vi "FormMain.vi"() -> ()   [LabVIEW 2013]
uses:
  S7Ref.vi
  resultShow.vi
panel:
  out "userStatus":string
  out "productsName 2":string
  out "takesTime":string
  out "rigStatus":string="提示信息"
  out "connectionMode":string
  out "productsName":string
  out "userName":string
  in  "VI引用句柄":refnum<vi>
  in  "复位":bool
  out "上序状态":string
  out "检具15":bool=TRUE
  out "扫码":bool
  in  "壳体码":string
  in  "countLeft":u32
  out "检具7":bool
  out "检具8":bool=TRUE
  in  "判定设定 2":string[][](table)
  in  "参数设定 2":string[][](table)
  out "表格控件":string[][](table)
  out "FFT范围 2":string[][](table)
  out "压力损失":bool
  out "外泄漏":bool
  out "检具9":bool
  out "检具10":bool=TRUE
  out "检具2":bool
  out "输出扭矩":dbl caption="数值 24" format="%.1f Nm"
  in  "打开按钮":bool
  in  "自动":bool
  out "检具1":bool=TRUE
  out "检具3":bool
  out "检具4":bool
  out "检具5":bool
  out "检具6":bool
  # "出厂检验台"
  # "步骤"
  # "完成计数："
  # "用时："
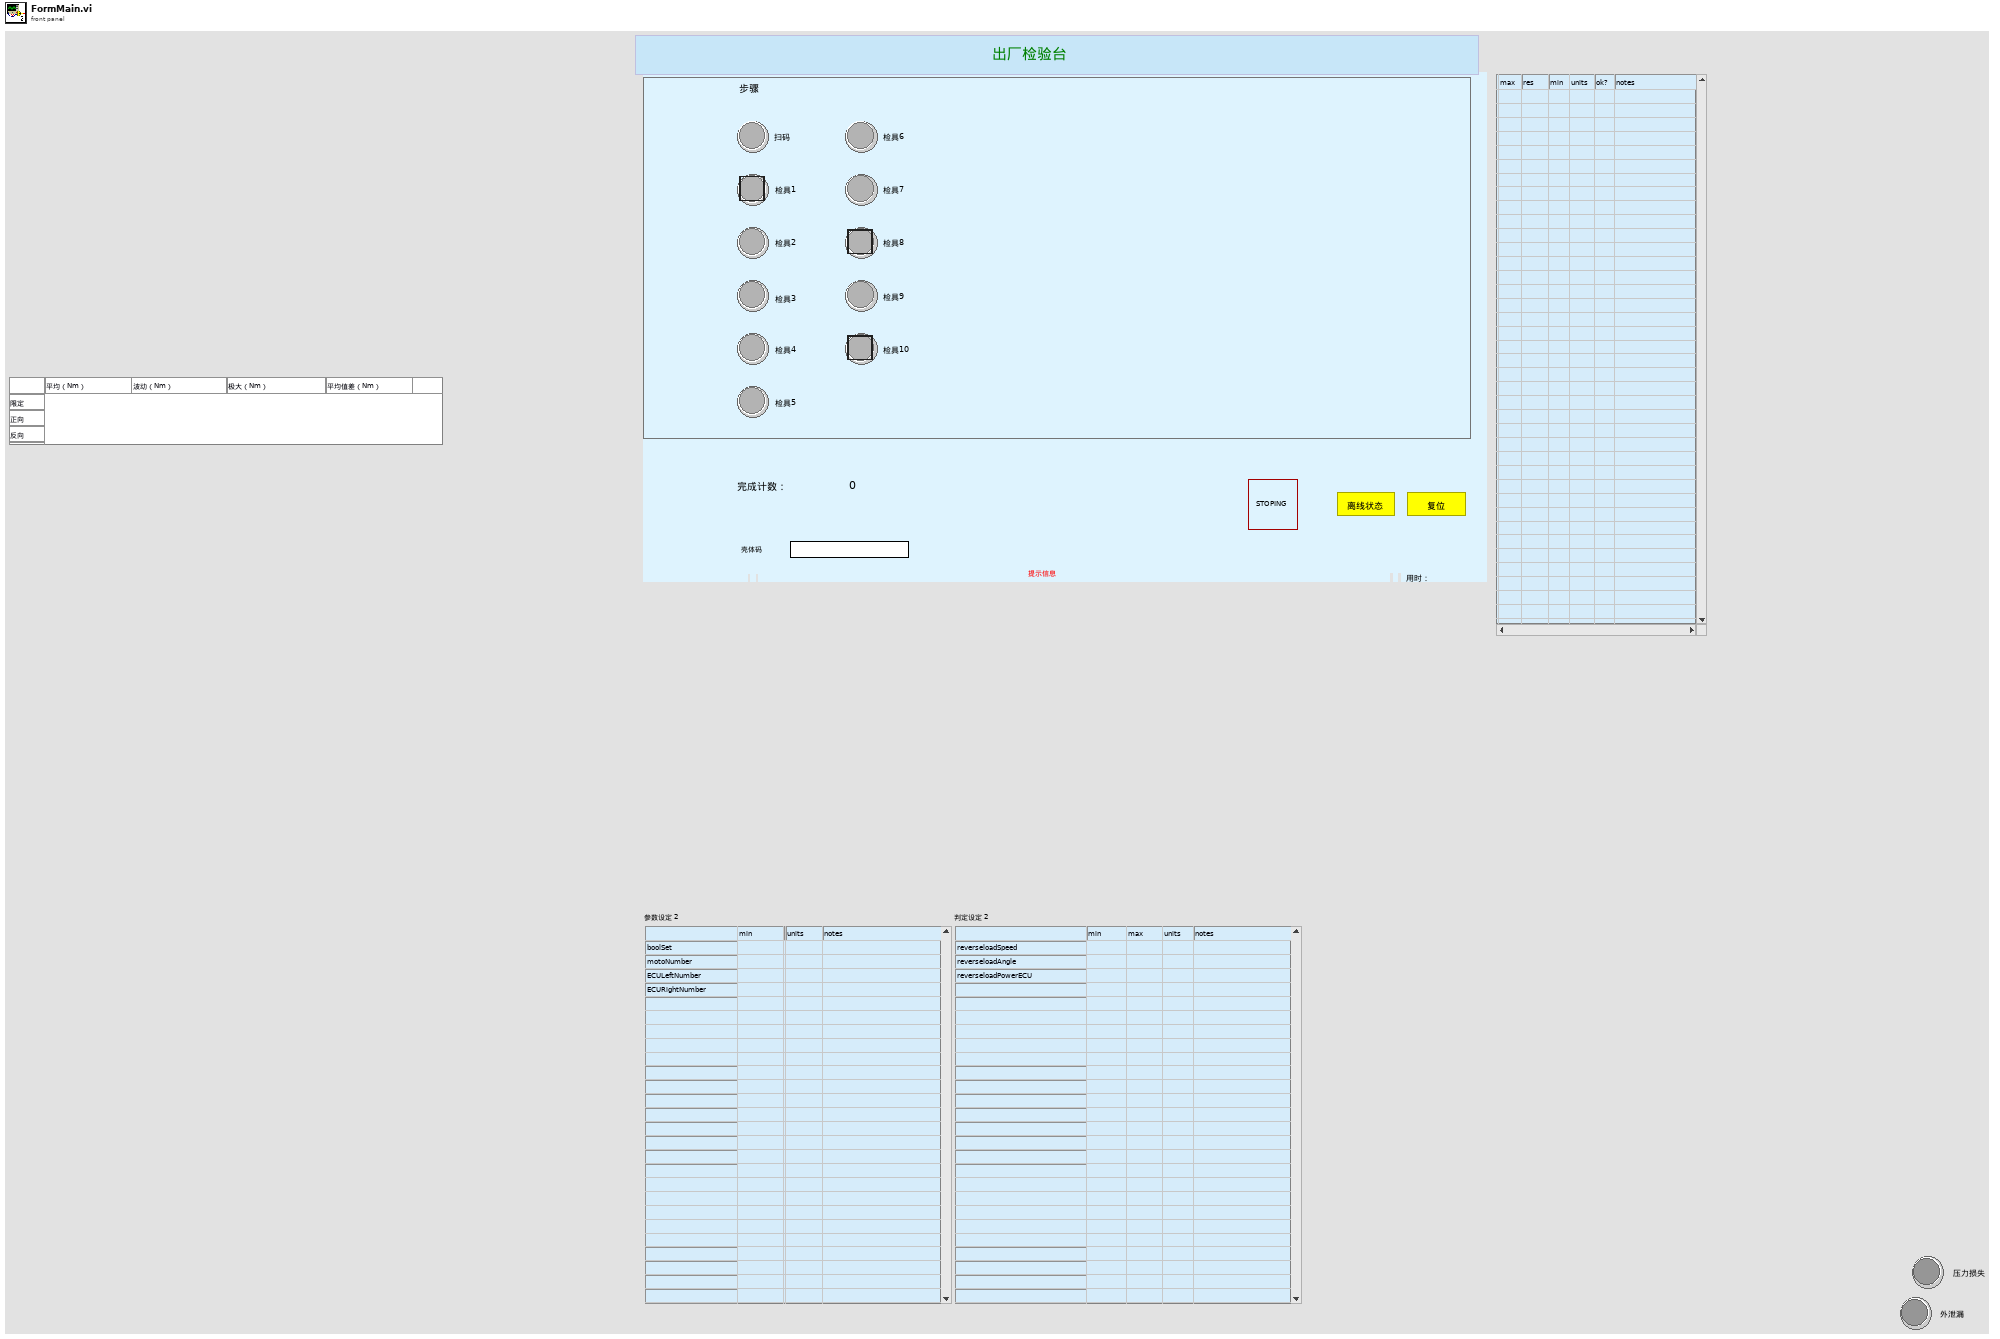
[diagram p1: front panel]
types:
  T1 = enum32{"Invalid", "Standard", "Closed", "Hidden", "Minimized", "Maximized"}
  T2 = cluster{"takesTime":refnum<vi>, "userStatus":refnum<vi>, "userName":refnum<vi>, "connectionMode":refnum<vi>, "productsName":refnum<vi>, "rigStatus":refnum<vi>, "壳体码":refnum<vi>, "上序状态":refnum<vi>}
  T3 = cluster{"userCode":string, "userName":string, "userStatus":string, "connectionMode":string}
  T4 = cluster{"Boolean array[0]":bool, "Boolean array[1]":bool, "Boolean array[2]":bool, "Boolean array[3]":bool, "Boolean array[4]":bool, "Boolean array[5]":bool, "Boolean array[6]":bool, "Boolean array[7]":bool, "Boolean array[8]":bool}
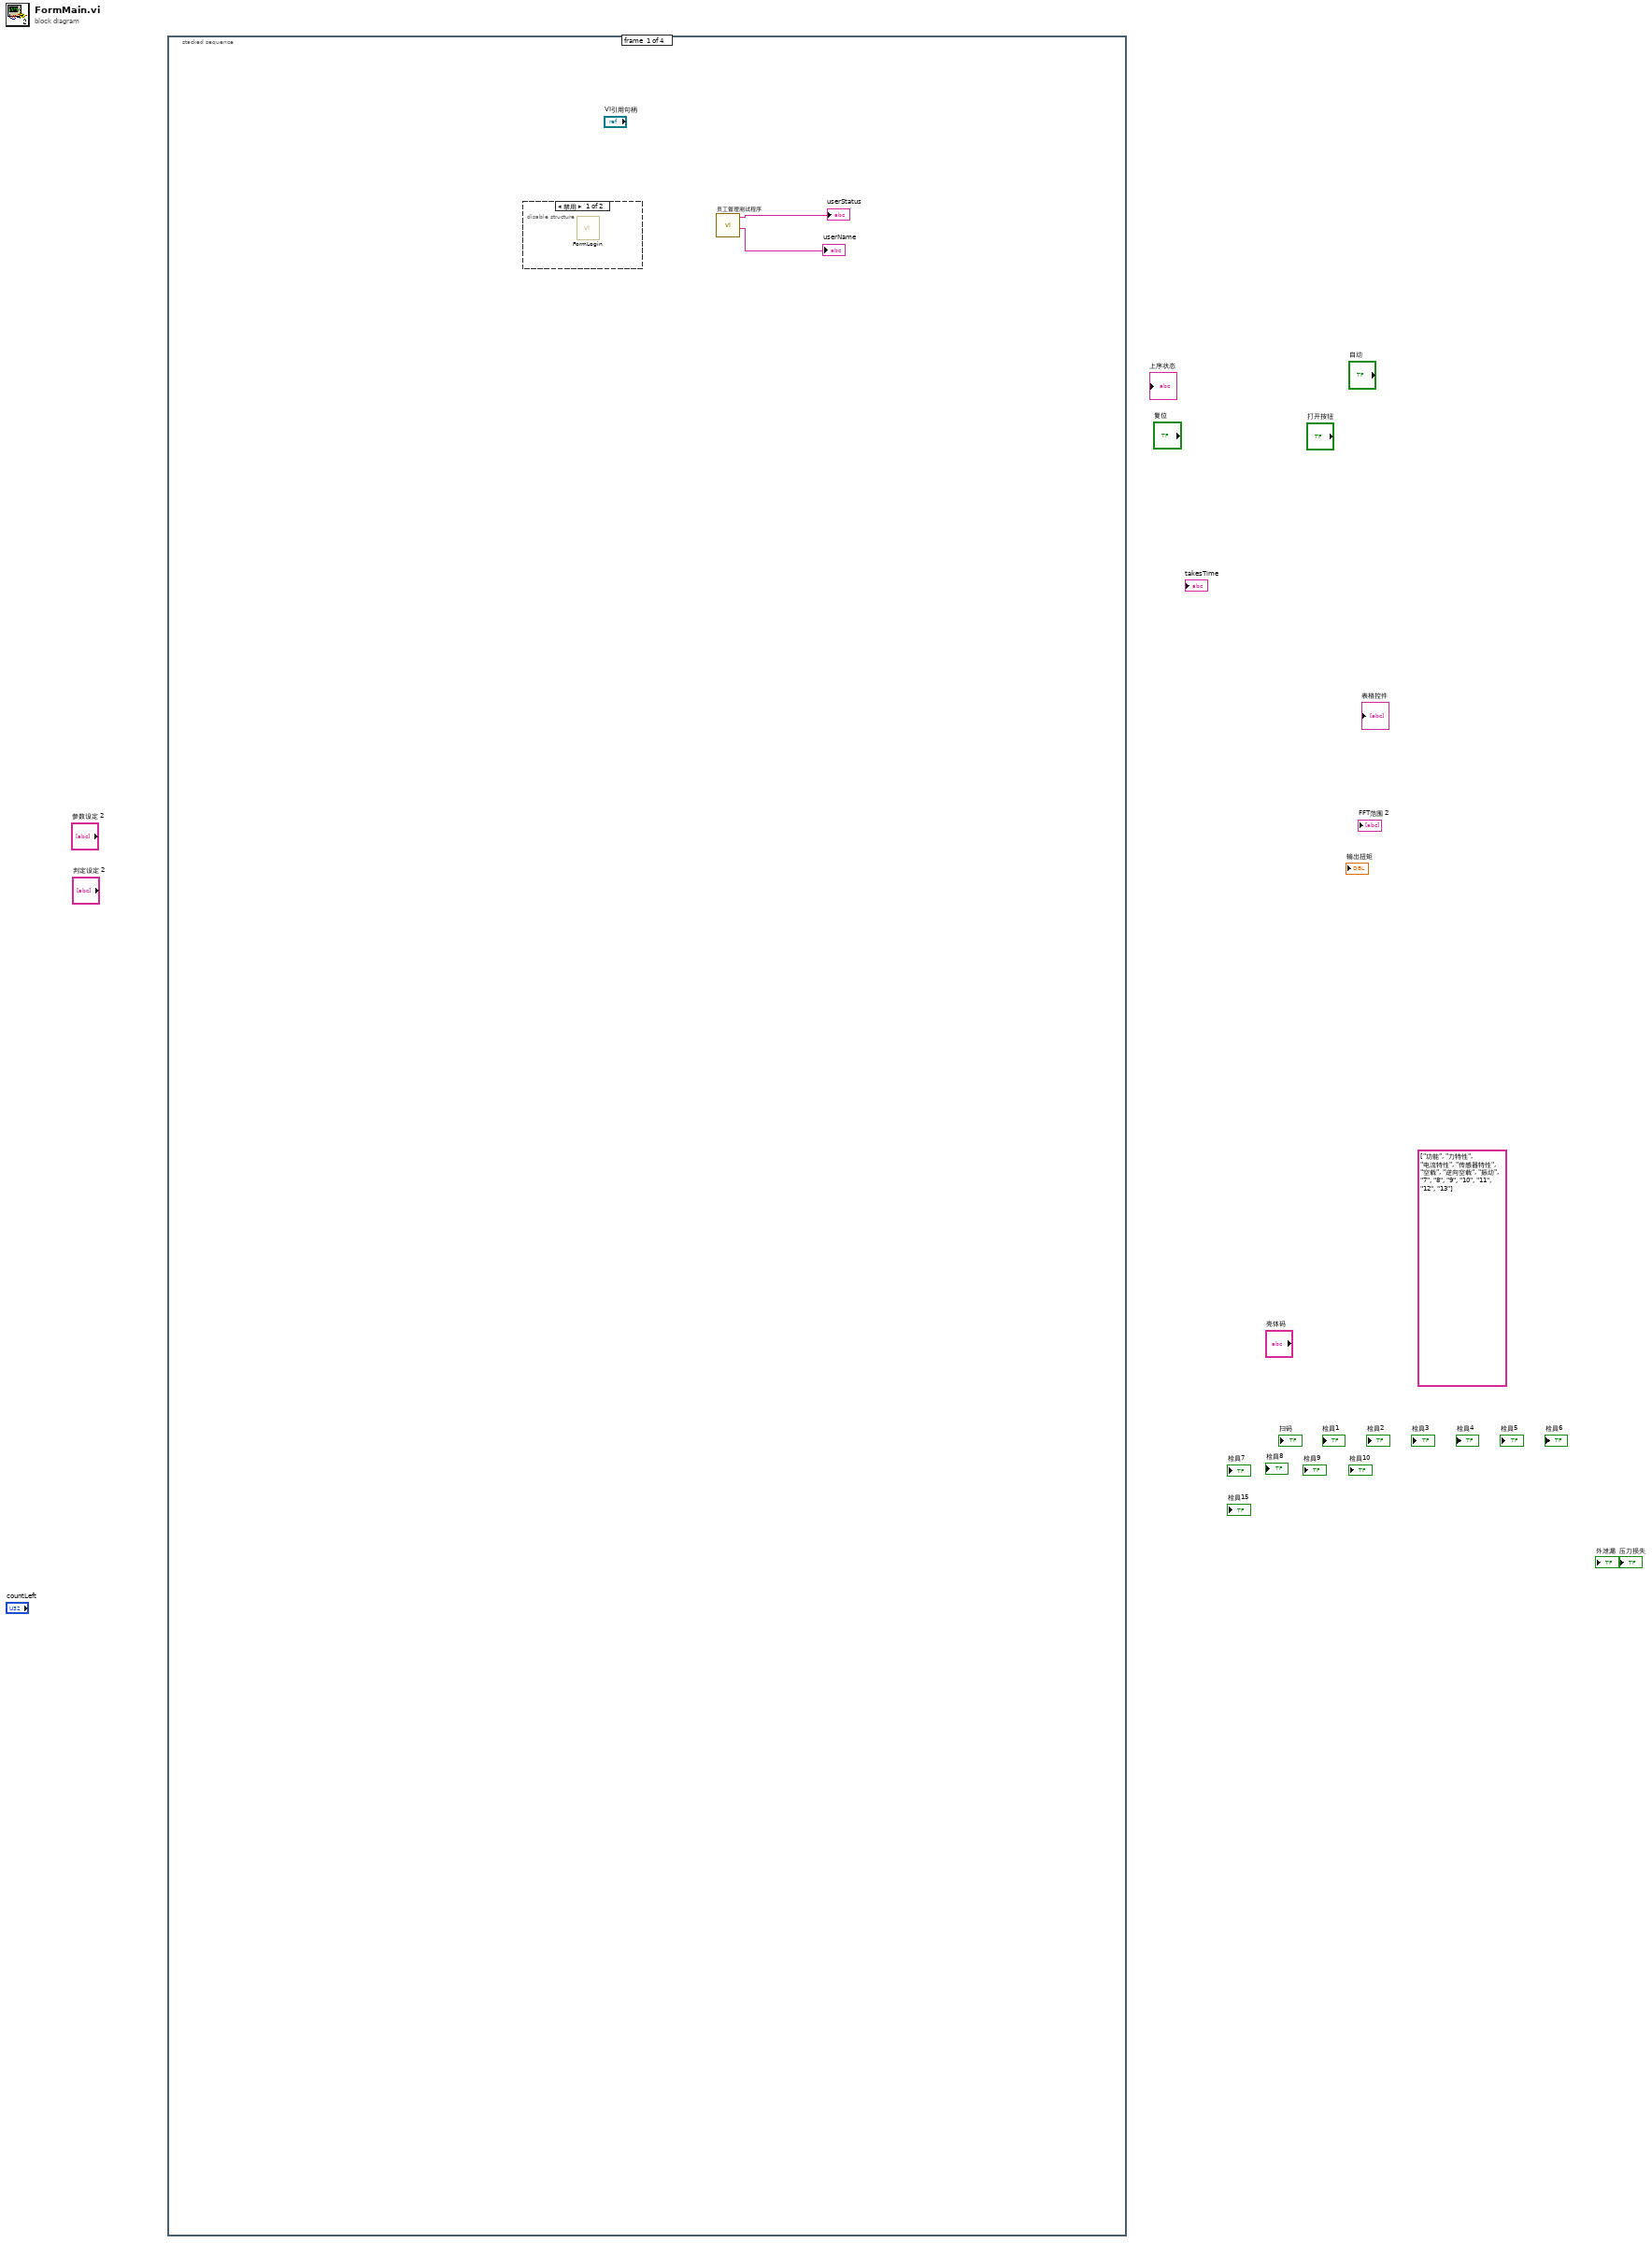
[diagram p0: block diagram]
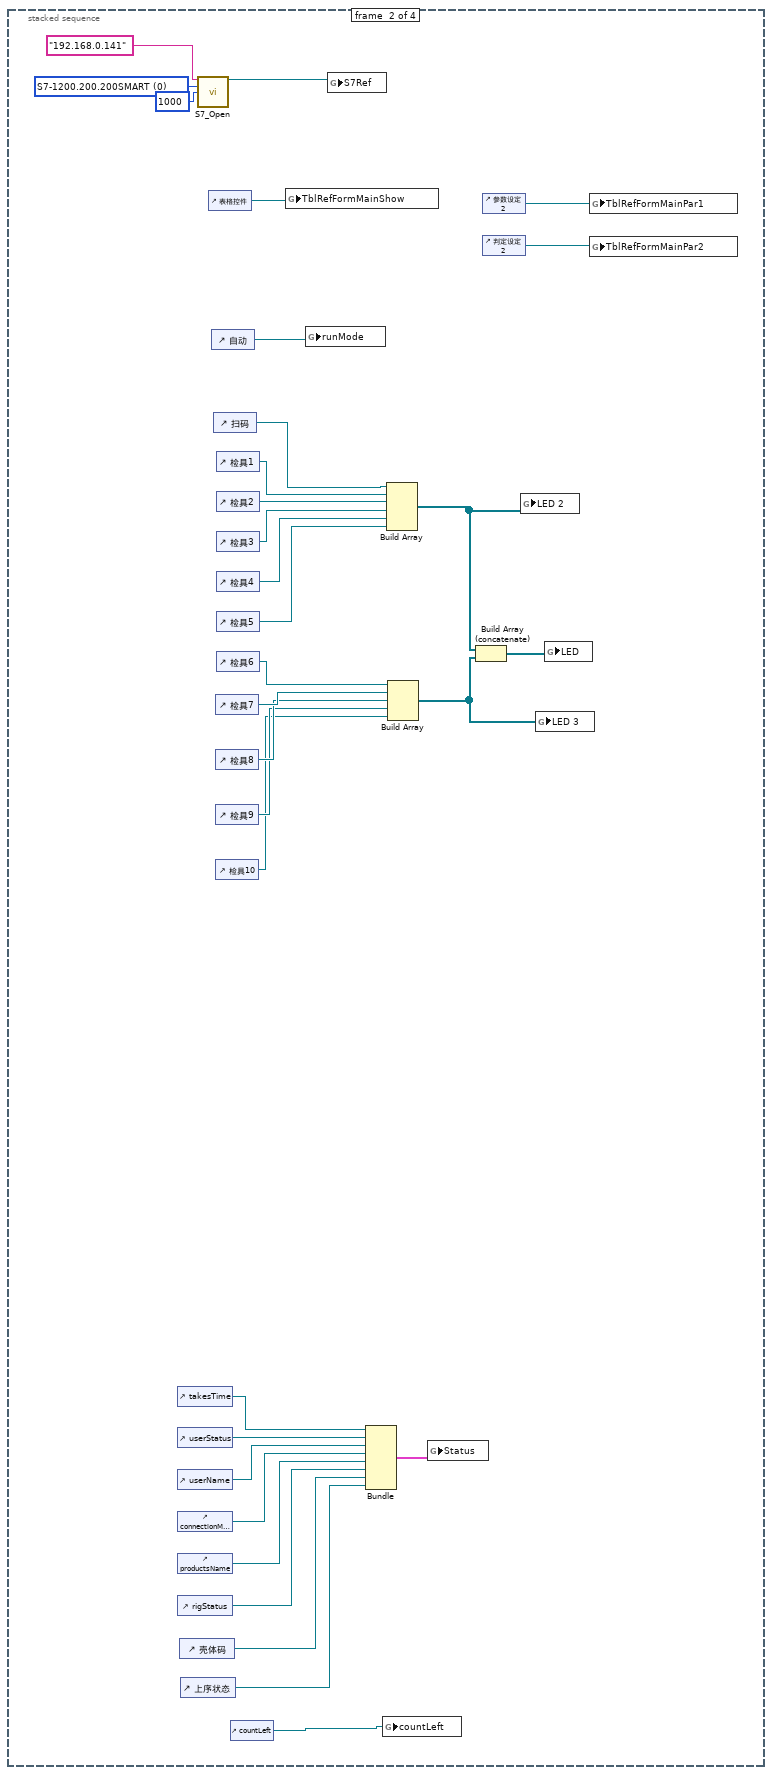
[diagram p3: hidden frame]
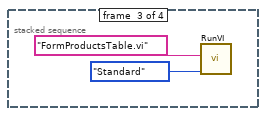
[diagram p4: hidden frame]
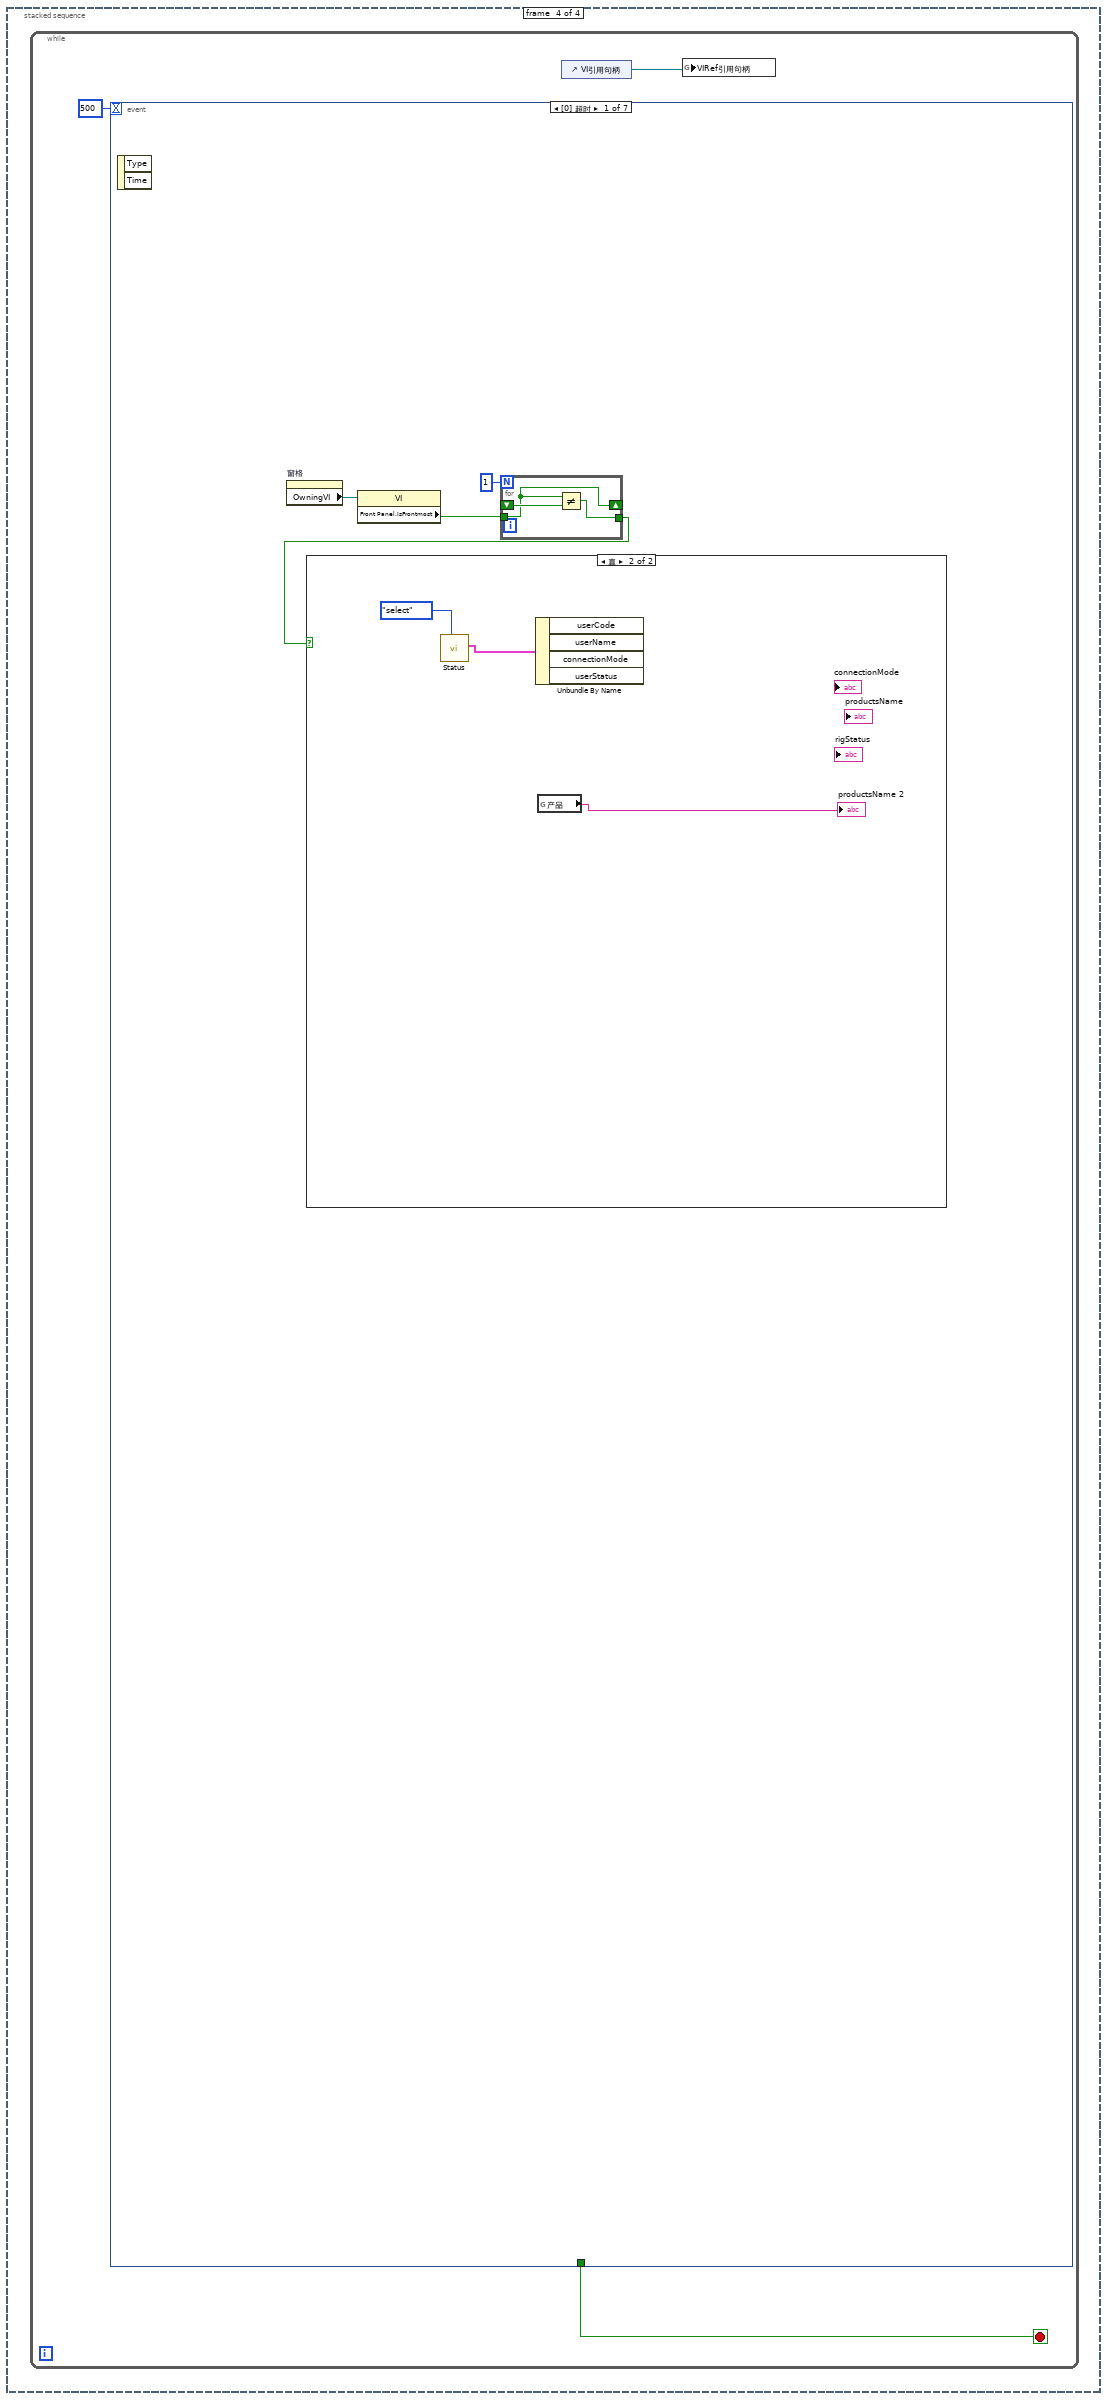
[diagram p5: hidden frame]
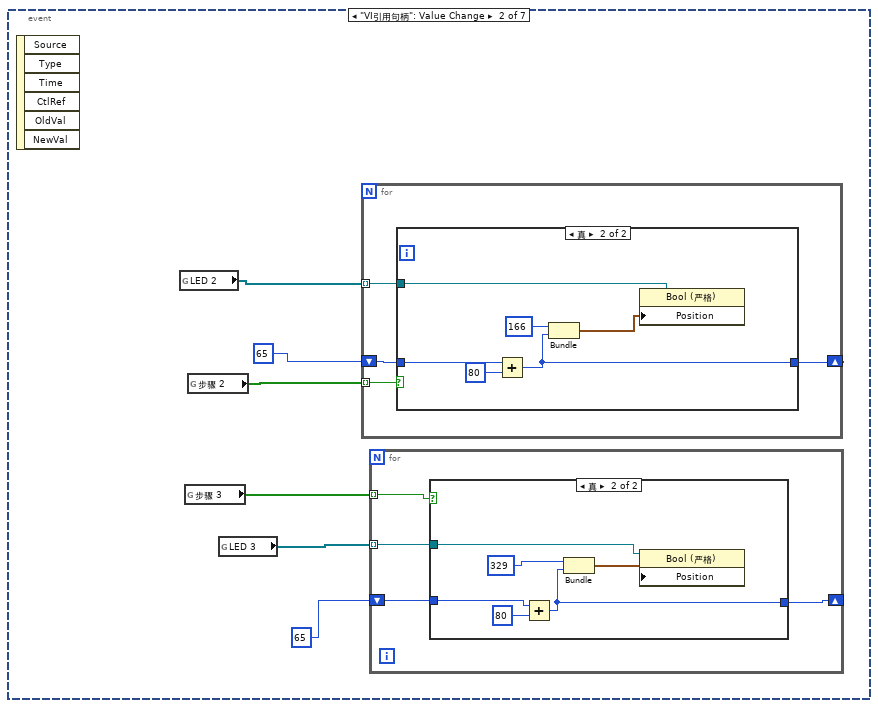
[diagram p7: hidden frame]
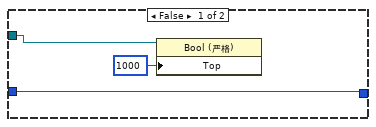
[diagram p8: hidden frame]
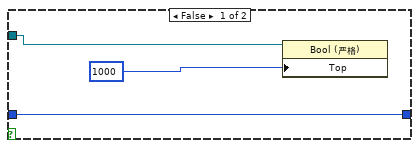
[diagram p9: hidden frame]
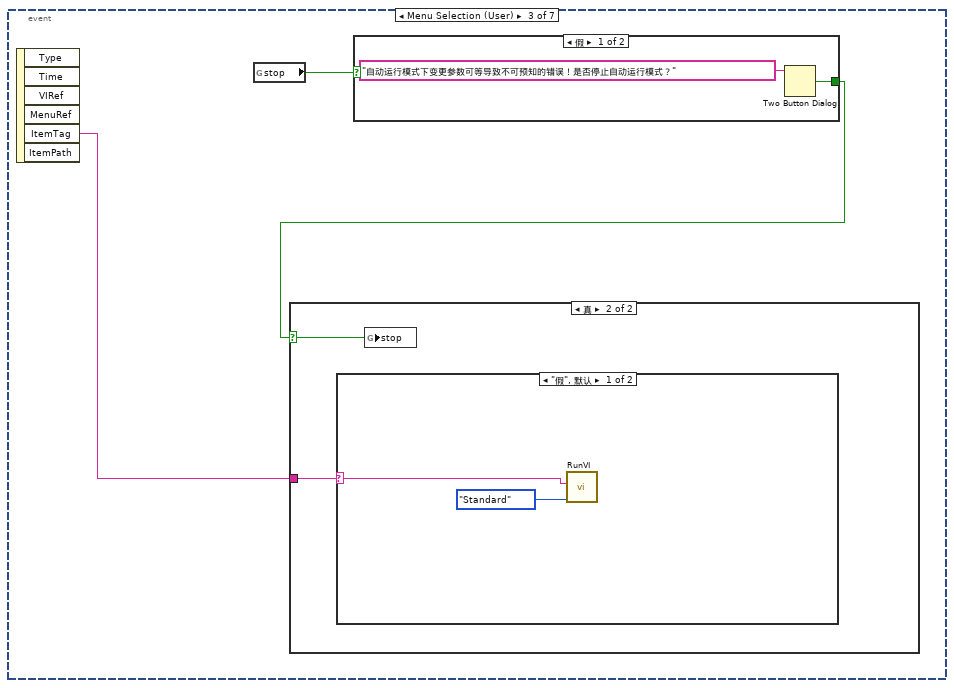
[diagram p10: hidden frame]
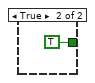
[diagram p11: hidden frame]
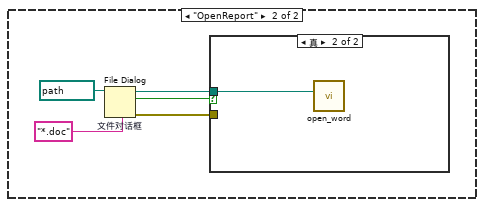
[diagram p13: hidden frame]
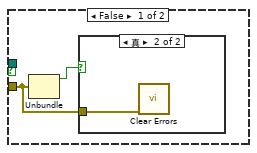
[diagram p14: hidden frame]
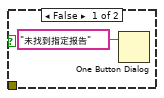
[diagram p15: hidden frame]
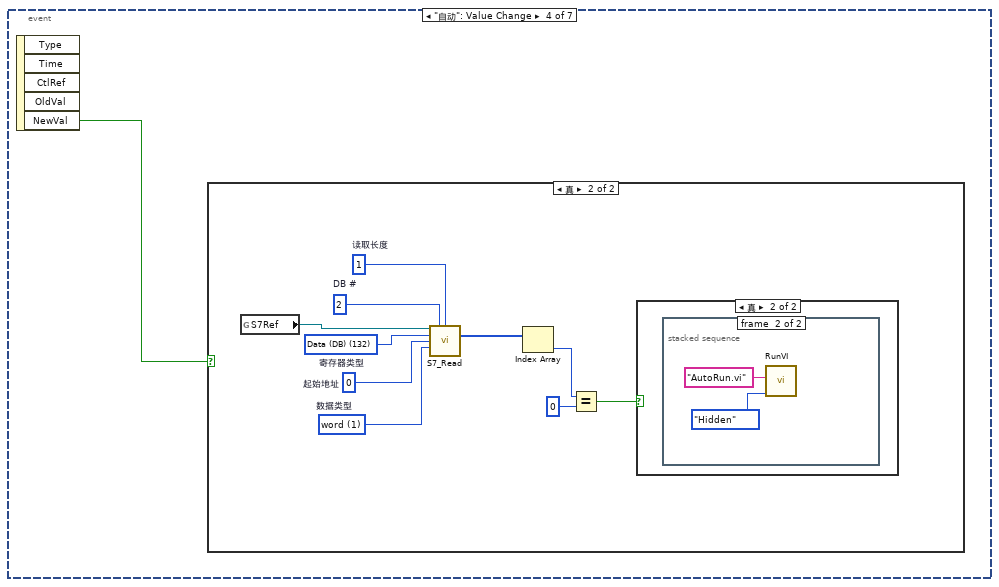
[diagram p16: hidden frame]
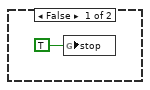
[diagram p17: hidden frame]
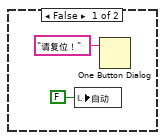
[diagram p18: hidden frame]
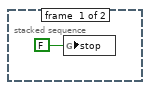
[diagram p19: hidden frame]
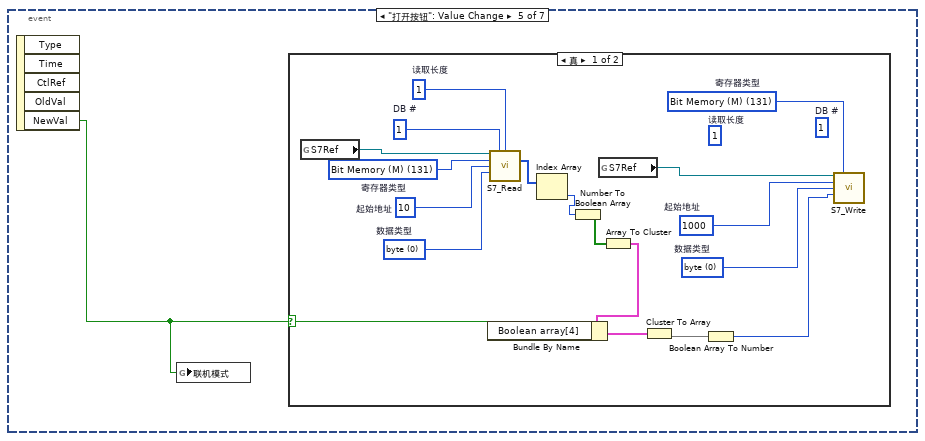
[diagram p20: hidden frame]
diagram:
  (unwired) string[] ["功能", "力特性", "电流特性", "传感器特性", "空载", "逆向空载", "振动", "7", "8", "9", "10", "11", "12", "13"] ("字符串[]")
  n1 = stacked-sequence {
    frame #0 {
      n2 = disable-structure shown="禁用" {
        frame Disabled {
          n3 = call "FormLogin.vi"() -> ()  [unwired: 12 in]
        }
        frame Enabled {
        }
      }
      n4 = call "员工管理测试程序.vi"() -> ("员工姓名"=→"userName":string, "员工ID"=→"userStatus":string)  [unwired: 10 in]
    }
    frame #1 {
      w32 = u8 0 items=["S7-1200.200.200SMART"=0, "S7-300"=2, "S7-400"=3] ("PLC 系列")
      n5 = control-ref of="takesTime"() -> (w17:refnum<vi>)
      n6 = control-ref of="userStatus"() -> (w23:refnum<vi>)
      n7 = control-ref of="userName"() -> (w22:refnum<vi>)
      n8 = control-ref of="connectionMode"() -> (w21:refnum<vi>)
      n9 = control-ref of="productsName"() -> (w20:refnum<vi>)
      n10 = control-ref of="rigStatus"() -> (w19:refnum<vi>)
      n11 = control-ref of="壳体码"() -> (w10:refnum<vi>)
      n12 = control-ref of="上序状态"() -> (w6:refnum<vi>)
      n13 = call "S7_Open.vi"("IP 地址"="192.168.0.141", "PLC 系列"=w32, "超时（MS）"=1000) -> ("TCP"=w30:refnum<k5>)  [unwired: 10 in, 2 out]
      n14 = control-ref of="表格控件"() -> (w34:refnum<vi>)
      n15 = control-ref of="自动"() -> (w29:refnum<vi>)
      n16 = control-ref of="扫码"() -> (w9:refnum<vi>)
      n17 = control-ref of="检具7"() -> (w13:refnum<vi>)
      n18 = control-ref of="检具8"() -> (w12:refnum<vi>)
      n19 = control-ref of="检具9"() -> (w8:refnum<vi>)
      n20 = control-ref of="检具10"() -> (w7:refnum<vi>)
      n21 = control-ref of="检具1"() -> (w24:refnum<vi>)
      n22 = control-ref of="检具2"() -> (w25:refnum<vi>)
      n23 = control-ref of="检具3"() -> (w26:refnum<vi>)
      n24 = control-ref of="检具4"() -> (w27:refnum<vi>)
      n25 = control-ref of="检具5"() -> (w28:refnum<vi>)
      n26 = control-ref of="检具6"() -> (w5:refnum<vi>)
      n27 = control-ref of="countLeft"() -> (w11:refnum<vi>)
      n28 = global write "resultShow.vi" "TblRefFormMainShow"(w34) -> ()
      n29 = global write "resultShow.vi" "runMode"(w29) -> ()
      n30 = global write "S7Ref.vi" "S7Ref"(w30) -> ()
      n31 = Bundle("takesTime"=w17, "userStatus"=w23, "userName"=w22, "connectionMode"=w21, "productsName"=w20, "rigStatus"=w19, "壳体码"=w10, "上序状态"=w6) -> (w18:T2)  [unwired: 1 in]
      n32 = global write "resultShow.vi" "countLeft"(w11) -> ()
      n33 = Build Array(w9, w24, w25, w26, w27, w28) -> (w4:refnum<vi>[])
      n34 = Build Array(w5, w13, w12, w8, w7) -> (w3:refnum<vi>[])
      n35 = global write "resultShow.vi" "Status"(w18) -> ()
      n36 = Build Array (concatenate)(w4, w3) -> (w14:refnum<vi>[])
      n37 = control-ref of="参数设定 2"() -> (w16:refnum<vi>)
      n38 = control-ref of="判定设定 2"() -> (w15:refnum<vi>)
      n39 = global write "resultShow.vi" "LED 2"(w4) -> ()
      n40 = global write "resultShow.vi" "LED 3"(w3) -> ()
      n41 = global write "resultShow.vi" "LED"(w14) -> ()
      n42 = global write "resultShow.vi" "TblRefFormMainPar1"(w16) -> ()
      n43 = global write "resultShow.vi" "TblRefFormMainPar2"(w15) -> ()
    }
    frame #2 {
      n44 = call "RunVI.vi"("状态"=T1."Standard", "名称或相对路径"="FormProductsTable.vi") -> ()  [unwired: 9 in, 1 out]
    }
    frame #3 {
      n45 = while {
        stop <- w39 stop-if-true
        n46 = event shown="[0] 超时" {
          selector: _ -> [_ _ _ _ _ _ _]
          dyn-events: _ -> [_ _ _ _ _ _ _]
          timeout: 500 -> [_ _ _ _ _ _ _]
          tunnel: [_ _ _ _ _ _ w159] -> w39
          event Timeout {
            n47 = event-data() -> ()  [unwired: 1 in, 2 out]
            n48 = property on="窗格" class="Pane"() -> ("OwningVI"=w43:refnum<vi>)  [unwired: 2 in, 2 out]
            n49 = property class="VI"(reference=w43) -> ("Front Panel.IsFrontmost"=w41:bool)  [unwired: 1 in, 2 out]
            n50 = for {
              N: 1 -> [_]
              shift-right: [w48] -> _
              shift-left: _ -> [w49]
              tunnel: w41 -> [w48]
              tunnel: [w47] -> w40
              n51 = Not Equal?(x=w48, y=w49) -> (x != y?=w47:bool)
            }
            n52 = case shown="真" w40 {
              frame False {
              }
              frame True {
                n53 = call "Status.vi"("模式"=enum16{"select", "insert", "update", "delete"}."select") -> ("元素"=w45:T3)  [unwired: 10 in]
                n54 = Unbundle By Name(w45) -> ()  [unwired: 4 out]
                n55 = global read "全局 3.vi" "产品"() -> (→"productsName 2":string)
              }
            }
          }
          event "VI引用句柄": Value Change {
            n56 = event-data() -> ()  [unwired: 1 in, 6 out]
            n57 = global read "resultShow.vi" "LED 2"() -> (w55:refnum<vi>[])
            n58 = global read "全局 3.vi" "步骤 3"() -> (w52:bool[])
            n59 = global read "全局 3.vi" "步骤 2"() -> (w53:bool[])
            n60 = global read "resultShow.vi" "LED 3"() -> (w51:refnum<vi>[])
            n61 = for {
              tunnel: w53 -> [w69] mode=indexing
              tunnel: w55 -> [w72] mode=indexing
              shift-right: [w70] -> _
              shift-left: 65 -> [w71]
              n62 = case shown="真" w69 {
                tunnel: w72 -> [w75 w81]
                tunnel: w71 -> [w73 w80]
                tunnel: [w73 w79] -> w70
                frame False {
                  n63 = property class="Bool (严格)"(reference=w75, "Top"=1000) -> ()  [unwired: 1 in, 2 out]
                }
                frame True {
                  n64 = Add(x=w80, y=80) -> (x+y=w79:i32)
                  n65 = Bundle(166, w79) -> (w78:cluster{i32, i32})  [unwired: 1 in]
                  n66 = property class="Bool (严格)"(reference=w81, "Position"=w78) -> ()  [unwired: 1 in, 2 out]
                }
              }
            }
            n67 = for {
              tunnel: w52 -> [w59] mode=indexing
              tunnel: w51 -> [w58] mode=indexing
              shift-right: [w56] -> _
              shift-left: 65 -> [w57]
              n68 = case shown="真" w59 {
                tunnel: w58 -> [w62 w65]
                tunnel: w57 -> [w61 w64]
                tunnel: [w61 w63] -> w56
                frame False {
                  n69 = property class="Bool (严格)"(reference=w62, "Top"=1000 ("位置:置顶")) -> ()  [unwired: 1 in, 2 out]
                }
                frame True {
                  n70 = Add(x=w64, y=80) -> (x+y=w63:i32)
                  n71 = Bundle(329, w63) -> (w67:cluster{i32, i32})  [unwired: 1 in]
                  n72 = property class="Bool (严格)"(reference=w65, "Position"=w67) -> ()  [unwired: 1 in, 2 out]
                }
              }
            }
          }
          event Menu Selection (User) {
            n73 = event-data() -> ("ItemTag"=w84:string)  [unwired: 1 in, 5 out]
            n74 = global read "全局 3.vi" "stop"() -> (w83:bool)
            n75 = case shown="假" w83 {
              tunnel: [w85 TRUE ("T button?")] -> w82
              frame False {
                n76 = Two Button Dialog(message="自动运行模式下变更参数可等导致不可预知的错误！是否停止自动运行模式？" ("消息")) -> (T button?=w85:bool)  [unwired: 2 in]
              }
              frame True {
              }
            }
            n77 = case shown="真" w82 {
              selector: w82 -> [_ w88]
              tunnel: w84 -> [_ w89]
              frame False {
              }
              frame True {
                n78 = case shown="\"假\", 默认" w89 {
                  selector: w89 -> [w90 _]
                  frame "假", Default {
                    n79 = call "RunVI.vi"("状态"=T1."Standard", "名称或相对路径"=w90) -> ()  [unwired: 9 in, 1 out]
                  }
                  frame "OpenReport" {
                    n80 = File Dialog "文件对话框"(6:"*.doc" ("prompt"), 11:path "D:/报表" ("开始路径")) -> (0:w92:errorcluster, 2:w94:bool, 3:w93:path)  [unwired: 1 in, 5 out]
                    n81 = case shown="真" w94 {
                      tunnel: w93 -> [_ w101]
                      tunnel: w92 -> [w97 _]
                      frame False {
                        n82 = Unbundle(w97) -> ("status"=w98:bool)  [unwired: 2 out]
                        n83 = case shown="真" w98 {
                          tunnel: w97 -> [_ w100]
                          frame False {
                            n84 = One Button Dialog(message="未找到指定报告" ("消息")) -> ()  [unwired: 1 in, 1 out]
                          }
                          frame True {
                            n85 = call <vilib>:"Clear Errors.vi"("error in (no error)"=w100) -> ()  [unwired: 6 in, 1 out]
                          }
                        }
                      }
                      frame True {
                        n86 = call "open_word.vi"("所选路径"=w101) -> ()  [unwired: 11 in]
                      }
                    }
                  }
                }
                n87 = global write "全局 3.vi" "stop"(w88) -> ()
              }
            }
          }
          event "自动": Value Change {
            n88 = event-data() -> ("NewVal"=w102:bool)  [unwired: 1 in, 4 out]
            n89 = case shown="真" w102 {
              frame False {
                n90 = global write "全局 3.vi" "stop"(TRUE ("布尔 1")) -> ()
              }
              frame True {
                w107 = u32 0  # 起始地址
                w109 = u16 1 items=["byte", "word", "Dword"]  # 数据类型
                w110 = u8 132 items=["I/O (P)"=128, "Input (I)"=129, "Output (Q)"=130, "Bit Memory (M)"=131, "Data (DB)"=132, "Instance Data (DI)"=133, "Local Data (L)"=134, "Predecessor Local Data (VL)"=135]  # 寄存器类型
                w111 = u16 1  # 读取长度
                w112 = u16 2  # DB #
                n91 = global read "S7Ref.vi" "S7Ref"() -> (w113:refnum<k5>)
                n92 = call "S7_Read.vi"("TCP"=w113, "DB #"=w112, "读取长度"=w111, "寄存器类型"=w110, "起始地址"=w107, "数据类型"=w109) -> ("数据"=w108:u32[])  [unwired: 6 in, 3 out]
                n93 = Index Array(array=w108) -> (element=w106:u32)  [unwired: 1 in]
                n94 = Equal?(x=w106, y=u32 0) -> (x = y?=w104:bool)
                n95 = case shown="真" w104 {
                  frame False {
                    n96 = local write "自动"(FALSE ("自动")) -> ()
                    n97 = One Button Dialog(message="请复位！" ("消息")) -> ()  [unwired: 1 in, 1 out]
                  }
                  frame True {
                    n98 = stacked-sequence {
                      frame #0 {
                        n99 = global write "全局 3.vi" "stop"(FALSE ("布尔 1")) -> ()
                      }
                      frame #1 {
                        n100 = call "RunVI.vi"("状态"=T1."Hidden", "名称或相对路径"="AutoRun.vi") -> ()  [unwired: 9 in, 1 out]
                      }
                    }
                  }
                }
              }
            }
          }
          event "打开按钮": Value Change {
            n101 = event-data() -> ("NewVal"=w119:bool)  [unwired: 1 in, 4 out]
            n102 = global write "resultShow.vi" "联机模式"(w119) -> ()
            n103 = case shown="真" w119 {
              selector: w119 -> [w134 w152]
              frame True {
                w128 = u32 10  # 起始地址
                w129 = u16 0 items=["byte", "word", "Dword"]  # 数据类型
                w130 = u8 131 items=["I/O (P)"=128, "Input (I)"=129, "Output (Q)"=130, "Bit Memory (M)"=131, "Data (DB)"=132, "Instance Data (DI)"=133, "Local Data (L)"=134, "Predecessor Local Data (VL)"=135]  # 寄存器类型
                w131 = u16 1  # 读取长度
                w132 = u16 1  # DB #
                w136 = u32 1000  # 起始地址
                w135 = u16 0 items=["byte", "word", "Dword"]  # 数据类型
                w120 = u8 131 items=["I/O (P)"=128, "Input (I)"=129, "Output (Q)"=130, "Bit Memory (M)"=131, "Data (DB)"=132, "Instance Data (DI)"=133, "Local Data (L)"=134, "Predecessor Local Data (VL)"=135]  # 寄存器类型
                (unwired) u16 1  # 读取长度
                (unwired) u16 1  # DB #
                n104 = global read "S7Ref.vi" "S7Ref"() -> (w133:refnum<k5>)
                n105 = call "S7_Read.vi"("TCP"=w133, "DB #"=w132, "读取长度"=w131, "寄存器类型"=w130, "起始地址"=w128, "数据类型"=w129) -> ("数据"=w127:u32[])  [unwired: 6 in, 3 out]
                n106 = Index Array(array=w127) -> (element=w126:u32)  [unwired: 1 in]
                n107 = Number To Boolean Array(number=w126) -> (Boolean array=w125:bool[])
                n108 = global read "S7Ref.vi" "S7Ref"() -> (w137:refnum<k5>)
                n109 = Array To Cluster(array=w125) -> (cluster=w124:T4)
                n110 = Bundle By Name(cluster=w124, "Boolean array[4]"=w134) -> (w123:T4)
                n111 = Cluster To Array(cluster=w123) -> (array=w122:bool[])
                n112 = Boolean Array To Number(Boolean array=w122) -> (number=w121:u32)
                n113 = call "S7_Write.vi"("TCP"=w137, "寄存器类型"=w120, "写入地址"=w136, "数据类型"=w135, "写入数据"=w121) -> ()  [unwired: 8 in, 3 out]
              }
              frame False {
                w146 = u32 10  # 起始地址
                w147 = u16 0 items=["byte", "word", "Dword"]  # 数据类型
                w148 = u8 131 items=["I/O (P)"=128, "Input (I)"=129, "Output (Q)"=130, "Bit Memory (M)"=131, "Data (DB)"=132, "Instance Data (DI)"=133, "Local Data (L)"=134, "Predecessor Local Data (VL)"=135]  # 寄存器类型
                w149 = u16 1  # 读取长度
                w150 = u16 1  # DB #
                w154 = u32 1000  # 起始地址
                w153 = u16 0 items=["byte", "word", "Dword"]  # 数据类型
                w138 = u8 131 items=["I/O (P)"=128, "Input (I)"=129, "Output (Q)"=130, "Bit Memory (M)"=131, "Data (DB)"=132, "Instance Data (DI)"=133, "Local Data (L)"=134, "Predecessor Local Data (VL)"=135]  # 寄存器类型
                (unwired) u16 1  # 读取长度
                (unwired) u16 1  # DB #
                n114 = global read "S7Ref.vi" "S7Ref"() -> (w151:refnum<k5>)
                n115 = call "S7_Read.vi"("TCP"=w151, "DB #"=w150, "读取长度"=w149, "寄存器类型"=w148, "起始地址"=w146, "数据类型"=w147) -> ("数据"=w145:u32[])  [unwired: 6 in, 3 out]
                n116 = Index Array(array=w145) -> (element=w144:u32)  [unwired: 1 in]
                n117 = Number To Boolean Array(number=w144) -> (Boolean array=w143:bool[])
                n118 = global read "S7Ref.vi" "S7Ref"() -> (w155:refnum<k5>)
                n119 = Array To Cluster(array=w143) -> (cluster=w142:T4)
                n120 = Bundle By Name(cluster=w142, "Boolean array[4]"=w152) -> (w141:T4)
                n121 = Cluster To Array(cluster=w141) -> (array=w140:bool[])
                n122 = Boolean Array To Number(Boolean array=w140) -> (number=w139:u32)
                n123 = call "S7_Write.vi"("TCP"=w155, "寄存器类型"=w138, "写入地址"=w154, "数据类型"=w153, "写入数据"=w139) -> ()  [unwired: 8 in, 3 out]
              }
            }
          }
          event "复位": Value Change {
            n124 = event-data() -> ("NewVal"=w156:bool)  [unwired: 1 in, 5 out]
            n125 = case shown="假" w156 {
              frame False {
                n126 = shared-variable "我的电脑\\Modbus.lvlib\\复位"(0) -> ()  [unwired: 1 in, 1 out]
              }
              frame True {
                n127 = shared-variable "我的电脑\\Modbus.lvlib\\复位"(1) -> ()  [unwired: 1 in, 1 out]
              }
            }
          }
          event Panel Close? {
            n128 = event-data() -> ()  [unwired: 1 in, 3 out]
            n129 = Two Button Dialog(message="真的要关闭程序吗？" ("消息")) -> (T button?=w160:bool)  [unwired: 2 in]
            n130 = case shown="真" w160 {
              tunnel: [FALSE w164] -> w159
              frame False {
              }
              frame True {
                n131 = stacked-sequence {
                  tunnel: [_ _ _ _ _ w172] -> w164
                  frame #0 {
                    n132 = for {
                      tunnel: string[] ["AutoRun.vi", "FormCamera.vi"] -> [w166] mode=indexing
                      n133 = call "CloseVI.vi"("名称或相对路径"=w166) -> ()  [unwired: 10 in, 1 out]
                    }
                  }
                  frame #1 {
                    n134 = shared-variable ".\\共享变量.lvlib\\string_5"("关闭程序中" ("string_5")) -> ()  [unwired: 1 in, 1 out]
                    n135 = global write "全局 3.vi" "stop"(TRUE ("布尔 2")) -> ()
                  }
                  frame #2 {
                    n136 = Wait (ms)(milliseconds to wait=u32 500 ("等待时间（毫秒）")) -> ()  [unwired: 1 out]
                  }
                  frame #3 {
                  }
                  frame #4 {
                    n137 = global read "S7Ref.vi" "S7Ref"() -> (w170:refnum<k5>)
                    n138 = call "S7_Close.vi"("TCP Connection Ref"=w170) -> ()  [unwired: 10 in, 1 out]
                  }
                  frame #5 {
                    w172 = TRUE
                    n139 = case shown="真" TRUE {
                      tunnel: w172 -> [_ w173]
                      frame False {
                      }
                      frame True {
                        n140 = Quit LabVIEW(quit? (T)=w173) -> ()
                      }
                    }
                  }
                }
              }
            }
            n141 = Not(x=w159) -> (.not. x?=w161:bool)
            n142 = event-data("Discard?"=w161) -> ()  [unwired: 1 in, 1 out]
          }
        }
        n143 = control-ref of="VI引用句柄"() -> (w37:refnum<vi>)
        n144 = global write "全局 3.vi" "VIRef引用句柄"(w37) -> ()
      }
    }
  }
